vi "Conversao_valores_engenharia_saida_TODOS.vi"(11 "todos_os_dados_SAIDA(Controle)":T1) -> (3 "todos_os_dados_SAIDA(Indicador)":T1)   [LabVIEW 2019]
uses:
  padrao_todos_os_dados_SAIDA.ctl
  padrao_UCM.004.EEL.0300_SAIDA.ctl
  padrao_UCM.004.EEL.0200_SAIDA.ctl
  padrao_INTERNO.ctl
  padrao_ADAM_SAIDA.ctl
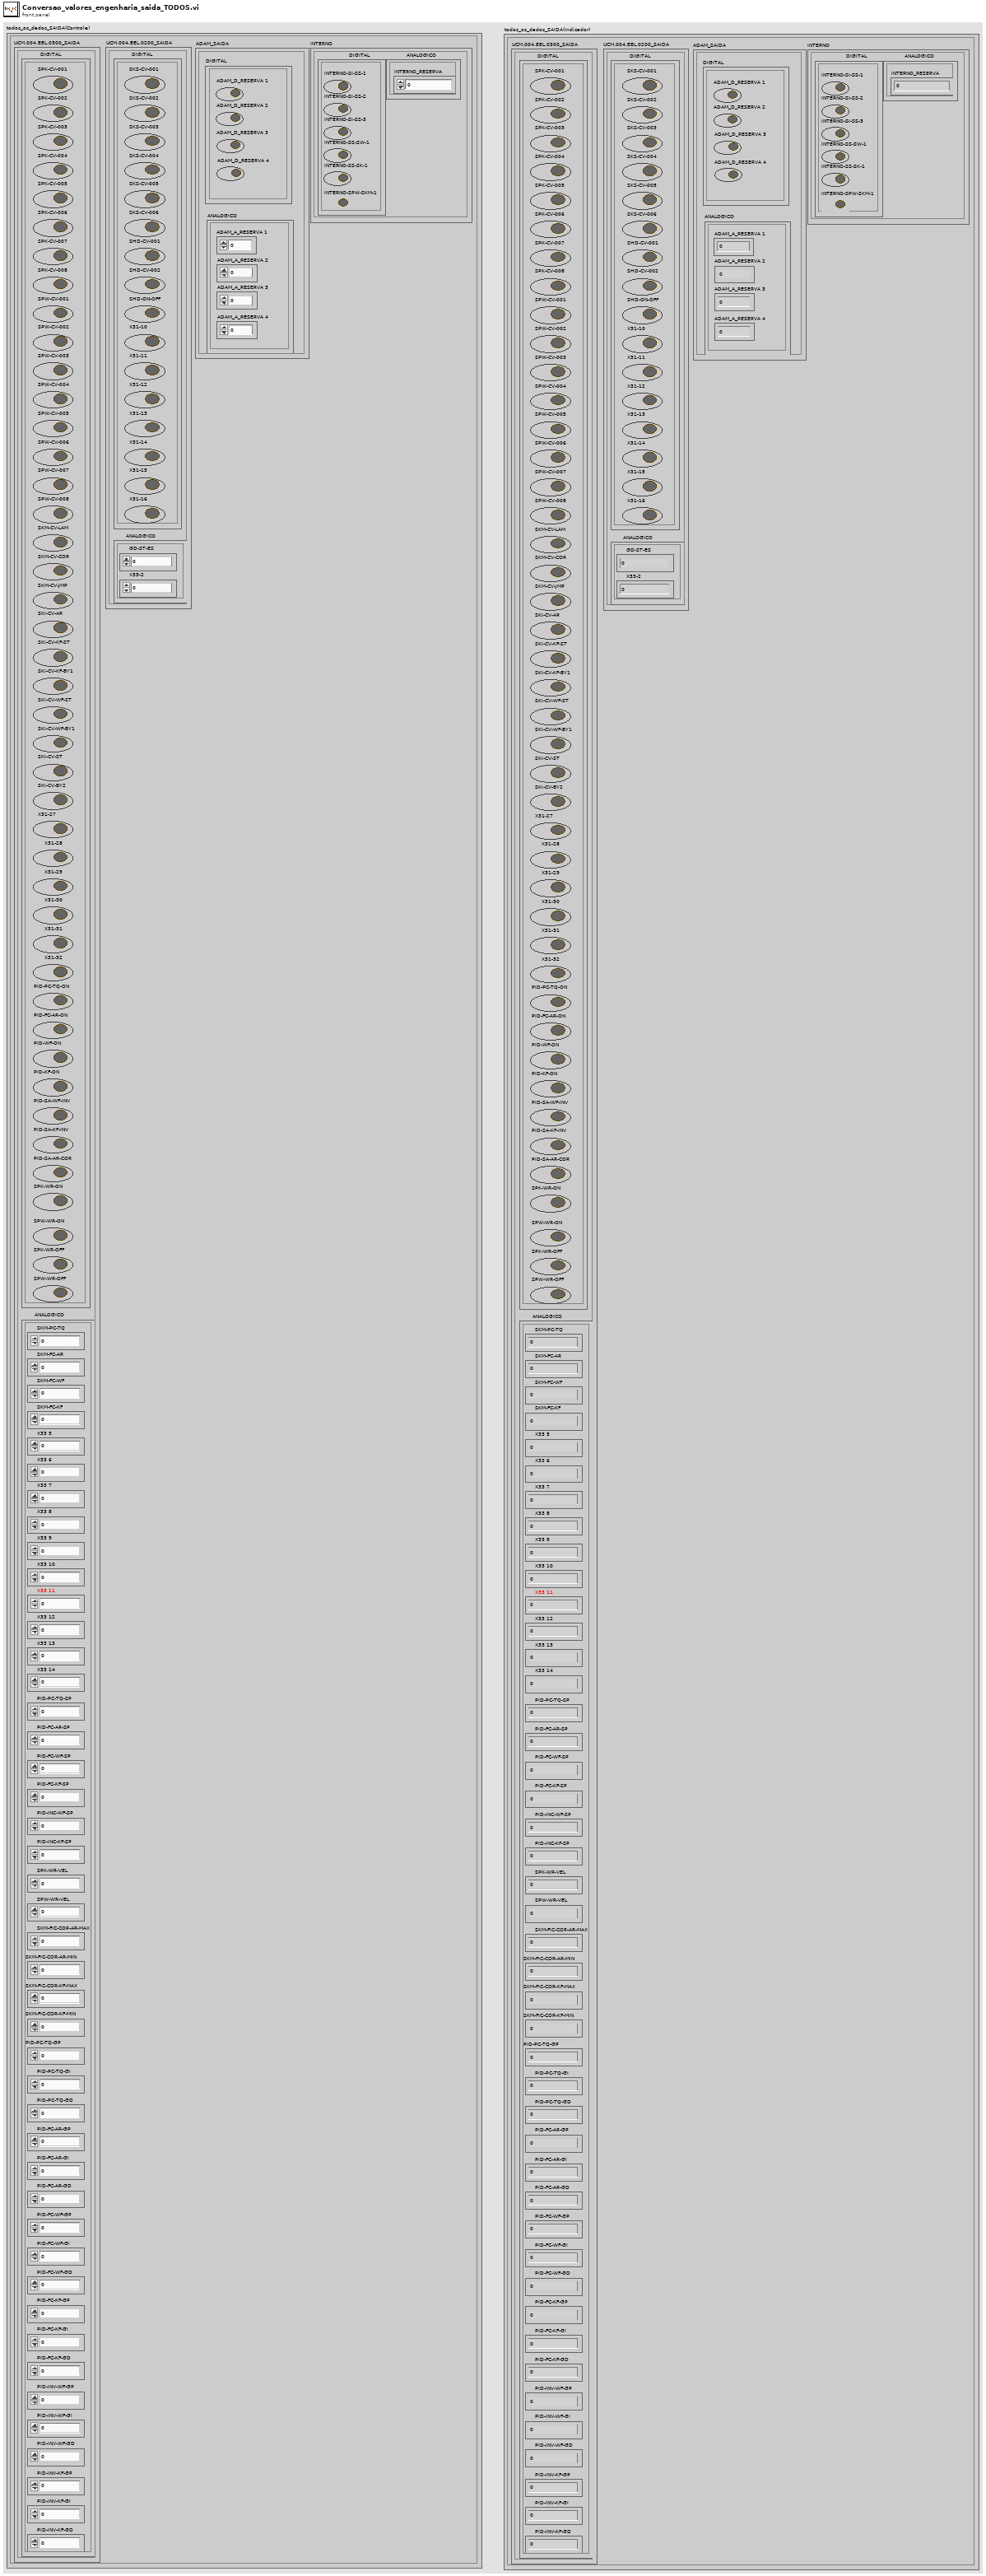
[diagram p1: front panel]
types:
  T1 = typedef "padrao_todos_os_dados_SAIDA.ctl" = cluster{"UCM.004.EEL.0300_SAIDA":T2, "UCM.004.EEL.0200_SAIDA":T3, "INTERNO":T4, "ADAM_SAIDA":T5}
  T2 = typedef "padrao_UCM.004.EEL.0300_SAIDA.ctl" = cluster{"DIGITAL":cluster{"SPK-CV-001":bool, "SPK-CV-002":bool, "SPK-CV-003":bool, "SPK-CV-004":bool, "SPK-CV-005":bool, "SPK-CV-006":bool, "SPK-CV-007":bool, "SPK-CV-008":bool, "SPW-CV-001":bool, "SPW-CV-002":bool, "SPW-CV-003":bool, "SPW-CV-004":bool, "SPW-CV-005":bool, "SPW-CV-006":bool, "SPW-CV-007":bool, "SPW-CV-008":bool, "SKM-CV-LAM":bool, "SKM-CV-COR":bool, "SKM-CV-JMP":bool, "SKI-CV-AR":bool, "SKI-CV-KF-ST":bool, "SKI-CV-KF-BY1":bool, "SKI-CV-WF-ST":bool, "SKI-CV-WF-BY1":bool, "SKI-CV-ST":bool, "SKI-CV-BY2":bool, "X31-27":bool, "X31-28":bool, "X31-29":bool, "X31-30":bool, "X31-31":bool, "X31-32":bool, "PID-PC-TQ-ON":bool, "PID-FC-AR-ON":bool, "PID-WF-ON":bool, "PID-KF-ON":bool, "PID-SA-WF-INV":bool, "PID-SA-KF-INV":bool, "PID-SA-AR-COR":bool, "SPK-WR-ON":bool, "SPW-WR-ON":bool, "SPK-WR-OFF":bool, "SPW-WR-OFF":bool}, "ANALOGICO":cluster{"SKM-PC-TQ":i16, "SKM-FC-AR":i16, "SKM-FC-WF":i16, "SKM-FC-KF":i16, "X33 5":i16, "X33 6":i16, "X33 7":i16, "X33 8":i16, "X33 9":i16, "X33 10":i16, "X33 11":i16, "X33 12":i16, "X33 13":i16, "X33 14":i16, "PID-PC-TQ-SP":i16, "PID-FC-AR-SP":i16, "PID-FC-WF-SP":i16, "PID-FC-KF-SP":i16, "PID-INC-WF-SP":i16, "PID-INC-KF-SP":i16, "SPK-WR-VEL":i32, "SPW-WR-VEL":i32, "SKM-FIC-COR-AR-MAX":dbl, "SKM-FIC-COR-AR-MIN":dbl, "SKM-FIC-COR-KF-MAX":dbl, "SKM-FIC-COR-KF-MIN":dbl, "PID-PC-TQ-GP":dbl, "PID-PC-TQ-GI":dbl, "PID-PC-TQ-GD":dbl, "PID-FC-AR-GP":dbl, "PID-FC-AR-GI":dbl, "PID-FC-AR-GD":dbl, "PID-FC-WF-GP":dbl, "PID-FC-WF-GI":dbl, "PID-FC-WF-GD":dbl, "PID-FC-KF-GP":dbl, "PID-FC-KF-GI":dbl, "PID-FC-KF-GD":dbl, "PID-INV-WF-GP":dbl, "PID-INV-WF-GI":dbl, "PID-INV-WF-GD":dbl, "PID-INV-KF-GP":dbl, "PID-INV-KF-GI":dbl, "PID-INV-KF-GD":dbl}}
  T3 = typedef "padrao_UCM.004.EEL.0200_SAIDA.ctl" = cluster{"DIGITAL":cluster{"SKS-CV-001":bool, "SKS-CV-002":bool, "SKS-CV-003":bool, "SKS-CV-004":bool, "SKS-CV-005":bool, "SKS-CV-006":bool, "SHD-CV-001":bool, "SHD-CV-002":bool, "SHD-ON-OFF":bool, "X31-10":bool, "X31-11":bool, "X31-12":bool, "X31-13":bool, "X31-14":bool, "X31-15":bool, "X31-16":bool}, "ANALOGICO":cluster{"GD-ST-ES":i16, "X33-2":i16}}
  T4 = typedef "padrao_INTERNO.ctl" = cluster{"DIGITAL":cluster{"INTERNO-SI-SS-1":bool, "INTERNO-SI-SS-2":bool, "INTERNO-SI-SS-3":bool, "INTERNO-SS-SW-1":bool, "INTERNO-SS-SK-1":bool, "INTERNO-SPW-SKM-1":bool}, "ANALOGICO":cluster{"INTERNO_RESERVA":dbl}}
  T5 = typedef "padrao_ADAM_SAIDA.ctl" = cluster{"DIGITAL":cluster{"ADAM_D_RESERVA 1":bool, "ADAM_D_RESERVA 2":bool, "ADAM_D_RESERVA 3":bool, "ADAM_D_RESERVA 4":bool}, "ANALOGICO":cluster{"ADAM_A_RESERVA 1":dbl, "ADAM_A_RESERVA 2":dbl, "ADAM_A_RESERVA 3":dbl, "ADAM_A_RESERVA 4":dbl}}
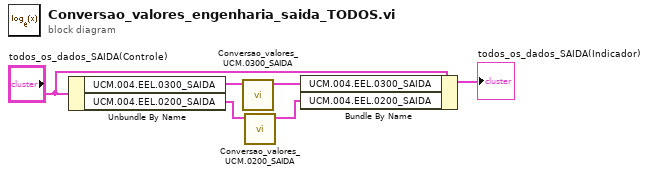
[diagram p0: block diagram]
diagram:
  n1 = Unbundle By Name("todos_os_dados_SAIDA(Controle)") -> ("UCM.004.EEL.0300_SAIDA"=w4:T2, "UCM.004.EEL.0200_SAIDA"=w2:T3)
  n2 = call "Conversao_valores_UCM.0300_SAIDA.vi"("UCM.004.EEL.0300_SAIDA(Controle)"=w4) -> ("UCM.004.EEL.0300_SAIDA(Indicador)"=w3:T2)  [unwired: 10 in]
  n3 = call "Conversao_valores_UCM.0200_SAIDA.vi"("UCM.004.EEL.0200_SAIDA(Controle)"=w2) -> ("UCM.004.EEL.0200_SAIDA(Indicador)"=w1:T3)  [unwired: 10 in]
  n4 = Bundle By Name(cluster="todos_os_dados_SAIDA(Controle)", "UCM.004.EEL.0300_SAIDA"=w3, "UCM.004.EEL.0200_SAIDA"=w1) -> (→"todos_os_dados_SAIDA(Indicador)":T1)
